vi "snr_recursive.vi"(8 "felharmonikus N":i32, 9 "width [Hz]":dbl=20.0, 11 "PSD":cluster{"f0":dbl, "df":dbl, "magnitude":dbl[]}(graph) caption="PSD IN") -> (0 "SNR":dbl, 1 "Noise Integral":dbl, 2 "Signal Integral":dbl, 3 "PSD":cluster{"f0":dbl, "df":dbl, "magnitude":dbl[]}[](graph))   [LabVIEW 2020]
panel:
  out "signal":cluster{"f0":dbl, "df":dbl, "magnitude":dbl[]}(graph)
  out "noise":cluster{"f0":dbl, "df":dbl, "magnitude":dbl[]}(graph)
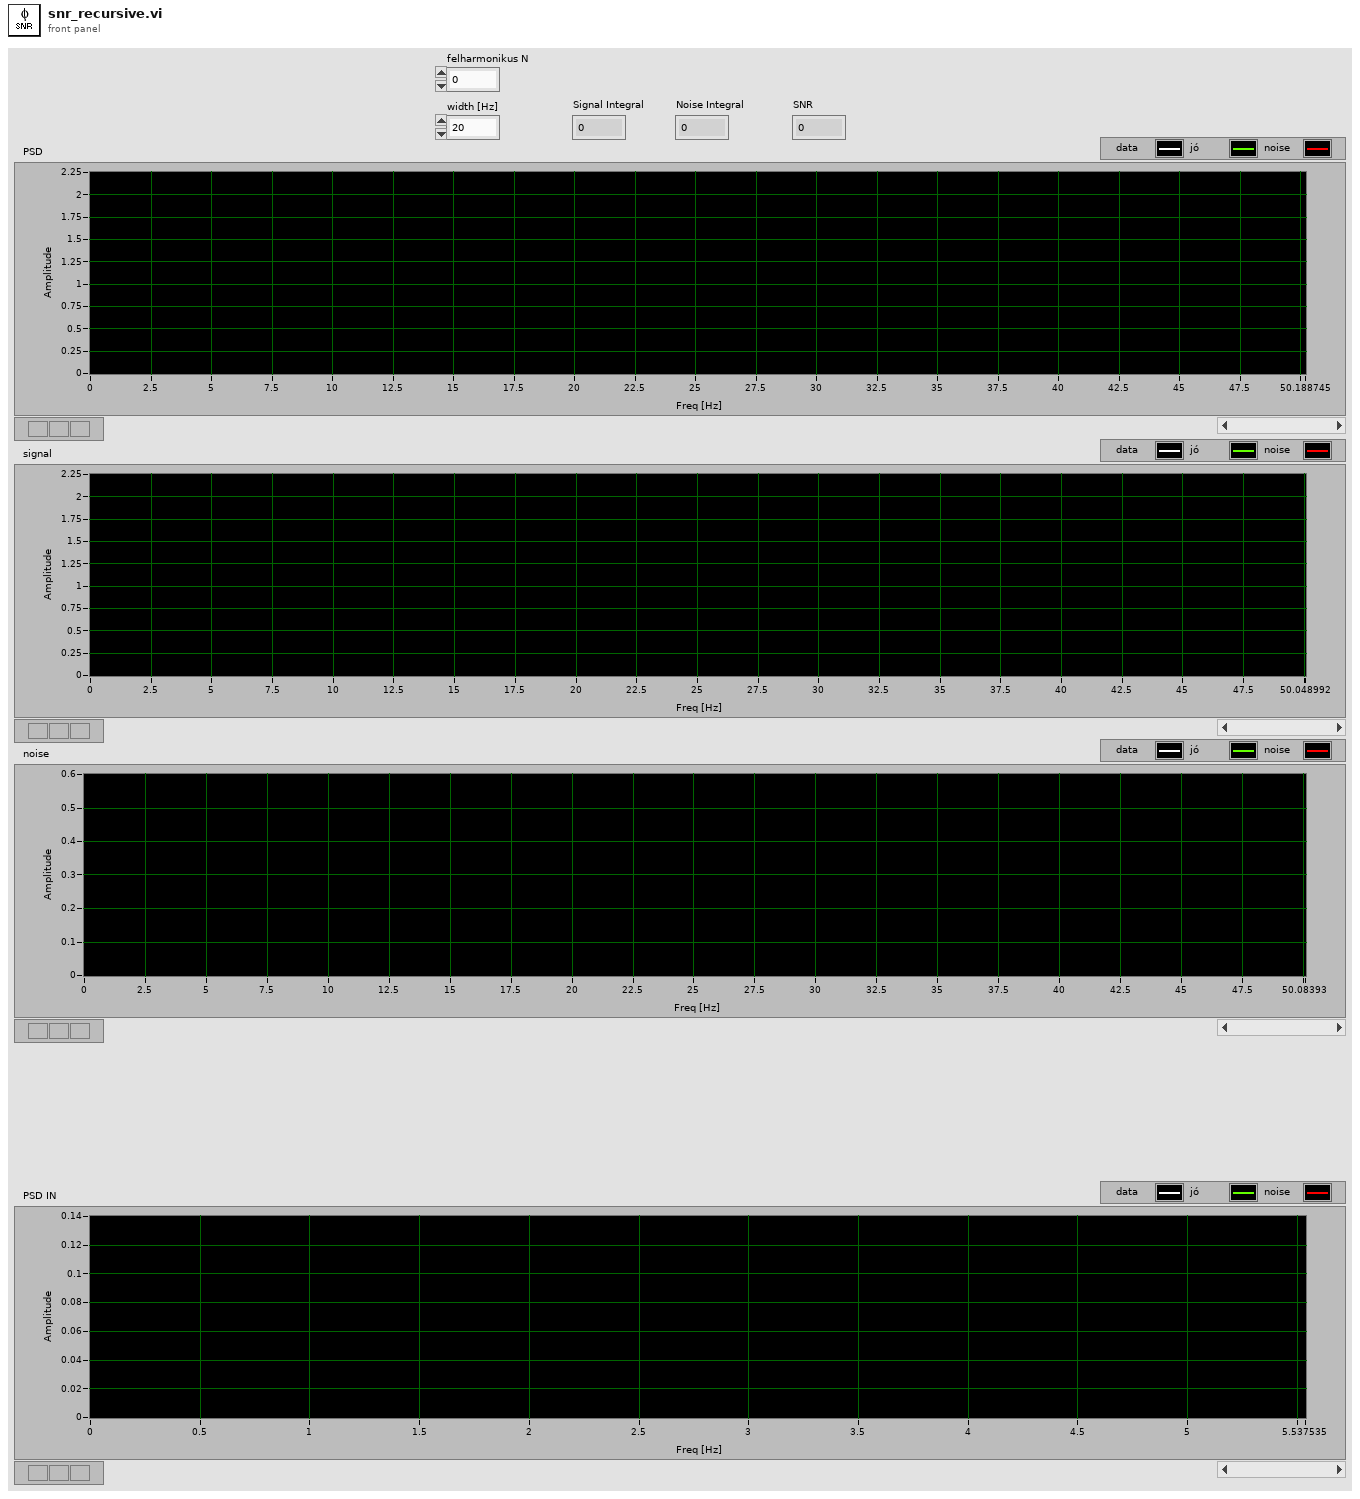
[diagram p1: front panel]
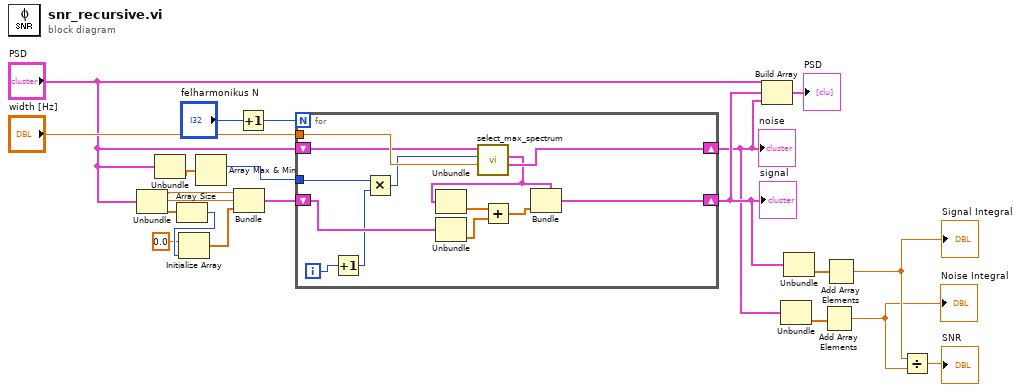
[diagram p0: block diagram]
diagram:
  n1 = Unbundle("PSD") -> ("f0"=w14:dbl, "df"=w13:dbl, "magnitude"=w12:dbl[])
  n2 = Unbundle("PSD") -> ("magnitude"=w2:dbl[])  [unwired: 2 out]
  n3 = Array Size(array=w12) -> (size(s)=w11:i32)
  n4 = Initialize Array(0.0 ("element"), w11) -> (w9:dbl[])
  n5 = Array Max & Min(array=w2) -> (max index (indices)=w1:i32)  [unwired: 3 out]
  n6 = Bundle("f0"=w14, "df"=w13, w9) -> (w8:cluster{"f0":dbl, "df":dbl, dbl[]})  [unwired: 1 in]
  n7 = Increment(x="felharmonikus N") -> (x+1=w7:i32)
  n8 = for {
    N: w7 -> [_]
    tunnel: "width [Hz]" -> [w29]
    shift-right: [w34] -> w3
    shift-left: "PSD" -> [w26]
    shift-right: [w30] -> w4
    shift-left: w8 -> [w27]
    tunnel: w1 -> [w24]
    i -> [w25]
    n9 = Increment(x=w25) -> (x+1=w23:i32)
    n10 = Multiply(x=w24, y=w23) -> (x*y=w22:i32)
    n11 = Unbundle(w27) -> (w32:dbl[])  [unwired: 2 out]
    n12 = call "select_max_spectrum.vi"("window freq"=w29, "index"=w22, "psd data"=w26) -> ("noise"=w34:cluster{"f0":dbl, "df":dbl, "magnitude":dbl[]}, "signal"=w28:cluster{"f0":dbl, "df":dbl, "magnitude":dbl[]})  [unwired: 6 in, 1 out]
    n13 = Unbundle(w28) -> ("magnitude"=w31:dbl[])  [unwired: 2 out]
    n14 = Add(x=w31, y=w32) -> (x+y=w33:dbl[])
    n15 = Bundle(cluster=w28, "magnitude"=w33) -> (w30:cluster{"f0":dbl, "df":dbl, "magnitude":dbl[]})  [unwired: 2 in]
  }
  "noise" <- w3
  "signal" <- w4
  n16 = Build Array("PSD", w4, w3) -> (→"PSD":cluster{"f0":dbl, "df":dbl, "magnitude":dbl[]}[])
  n17 = Unbundle(w3) -> ("magnitude"=w17:dbl[])  [unwired: 2 out]
  n18 = Unbundle(w4) -> (w16:dbl[])  [unwired: 2 out]
  n19 = Add Array Elements(numeric array=w17) -> (sum=w18:dbl)
  "Noise Integral" <- w18
  n20 = Add Array Elements(numeric array=w16) -> (sum=w19:dbl)
  "Signal Integral" <- w19
  n21 = Divide(x=w19, y=w18) -> (x/y=→"SNR":dbl)
